vi "RT_Velocity mode_Oct 25.vi"() -> ()   [LabVIEW 2018]
uses:
  <vilib>/Platform/TimedLoop/XDataNode/XDataNode.xnode
  <vilib>/Platform/TimedLoop/XDataNode/nitl_modes.ctl
  <vilib>/Platform/TimedLoop/XDataNode/XDNodeRunTimeDep.lvlib
  <vilib>/Platform/TimedLoop/XDataNode/wakeup.ctl
  <vilib>/Platform/TimedLoop/XDataNode/timing_clust.ctl
  <vilib>/rvi/interface/nirviReadWriteControl/nirviReadWriteControl.xnode
  NiFpgaLv.dll
  <vilib>/Utility/error.llb/Error Cluster From Error Code.vi
  <vilib>/rvi/interface/Simulation/niFpgaSimulationCallBeginRW.vi
  <vilib>/rvi/errors/niLvFpgaAdjustHostInterfaceError.vi
  <vilib>/rvi/interface/nirviOpenFPGA/nirviOpenFPGA.xnode
  Type Defs/BL Measurement States.ctl
  <vilib>/rvi/interface/nirviCloseFPGA/nirviCloseFPGA.xnode
  <vilib>/FPGAPlugInAG/Dynamic/niLvFpga_Close_Dynamic.vi
  UNCC Watt balance Oct19/FPGA Bitfiles/UNCCWattbalanceO_FPGATarget_fpganestedFORW&R_sb-Oe1PDHtY.lvbitx
  FPGA files/fpga_nestedFOR_W&R_ADC_W_2DACs_Write_then_CLK.vi
  <vilib>/FPGAPlugInAG/myRIO-1900/niLvFpga_Open_myRIO-1900.vi
  <vilib>/rvi/interface/common/dynamic/niFpgaDynamicAddResources.vi
  <vilib>/addons/control/pid/NI_PID_pid.lvlib
  <vilib>/addons/control/pid/pid.llb/PID Lead-Lag (DBL).vi
panel:
  out "Velocity (m/s)":dbl=0.03333406380742028
  out "BL":dbl=14.310883864096947
  out "Cycles 2":dbl=2.5
  out "Time period 2":dbl=0.03704 format="%.4f"
  out "Amplitude (EMF)":dbl=0.47703991586638894 format="%.6f"
  out "Cycles":dbl=2.0
  out "Time period":dbl=0.037 format="%.4f"
  out "Amplitude (CP)":dbl=0.0001964918899367253 format="%.6f"
  in  "no. data points":u16=500
  in  "Measure":bool
  in  "Period (us)":i64=200
  in  "EMF Gain":dbl=1.0
  in  "offset (V)":dbl format="%#_13g"
  in  "frequency (Hz)":dbl=27.0 format="%#_13g"
  in  "amplitude (V)":dbl=0.4 format="%#_13g"
  out "Late? [i-1]":bool
  in  "Stop Button":bool
  out "?":cluster{dbl, dbl}(graph)={161.59573981109904, -162.80879503181404}
  out "sine fit debug":dbl[][](graph)=[[5.264201901216106e-07, 8.666859941712313e-06, 1.4091276683400212e-05, 2.2193570044402394e-05, 2.7587469673619477e-05, 3.5636358087797725e-05, 4.0946335657720054e-05, 4.886552634389733e-05, 5.410684041076032e-05, 6.187344553458349e-05, 6.953324076475882e-05, 7.45838228786792e-05, 8.20605154340296e-05, 8.694325342936049e-05, 9.181073286845596e-05, 9.892122007415655e-05, 0.00010359033828219172, 0.00011045668858812577, 0.00011494270412133601, 0.000121526771136915, 0.0001257915376047118, 0.0001320551749393472, 0.00013609869234173057, 0.00014198086577048074, 0.0001457726169949799, 0.00015131147290843336, 0.00015482857012069515, 0.00015994018645955715, 0.00016319788821581697, 0.00016785937714573442, 0.0001708500541678746, 0.00017506141568884748, 0.00017772403375192634, 0.00018147763858583694, 0.00018381982696797223, 0.0001871156751148206, 0.00018912980453789457, 0.000191906861772739, 0.0001936005615148694, 0.00019586645711582766, 0.0001978271815920777, 0.00019896394403161566, 0.00019994812090879955, 0.00020119169324198536, 0.00020184781116010795, 0.0002025573340250545, 0.00020285487587164497, 0.00020303797854646986, 0.00020299983215588135, 0.00020264125608434924, 0.000202259792178464, 0.00020139768375116338, 0.00020063475593939294, 0.00019926911515632384, 0.0001981857576636098, 0.00019629369669041909, 0.00019489753879487918, 0.00019249431618780224, 0.0001907395822207302, 0.00018787097364847332, 0.0001857958100004577, 0.00018243892762866772, 0.0001800433342997085, 0.00017622869524085627, 0.00017351267223095345, 0.00016924790576315664, 0.00016625722874101648, 0.0001615423348642751, 0.00015660619192212028, 0.00015315775821291784, 0.00014780200497428928, 0.00014409417580908492, 0.00014028716602835034, 0.00013441262187771787, 0.0001303614751972168, 0.0001241207256969345, 0.0001198407006729023, 0.00011328715076979413, 0.00010880113523658388, 0.00010191952637441442, 9.724277888826156e-05, 9.008651601385474e-05, 8.522666585287697e-05, 7.781863680058592e-05, 7.282145963348946e-05, 6.518455223766725e-05, 6.003478950821672e-05, 5.224529655004042e-05, 4.697346537070661e-05, 3.903901612829393e-05, 3.101301554846879e-05, 2.561148664113401e-05, 2.024047484627004e-05, 1.2100035094679337e-05, 6.6679890748737334e-06, -1.4800799548346732e-06, -6.919755252757983e-06, -1.5044936448113276e-05, -2.044646535544806e-05, -2.8472465935273197e-05, -3.377481422707782e-05, -4.166348780078428e-05, -4.685902619894104e-05, -5.456459709782259e-05, -5.962280848986067e-05, -6.71223888795642e-05, -7.20356439873659e-05, -7.928345819918517e-05, -8.404412774463277e-05, -9.10401757785678e-05, -9.56253719273082e-05, -0.00010233150739277047, -0.00010673360086668595, -0.00011311167737308692, -0.00011726963394723587, -0.00012332728077269324, -0.00012724872972519338, -0.00013294017120100092, -0.0001366327418099699, -0.0001419122022674214, -0.0001453148603079176, -0.00015019759830324852, -0.00015331797305338964, -0.00015774295436165825, -0.00016192379877016033, -0.00016455589972076836, -0.00016705067366525774, -0.00017056777087751953, -0.00017274974441918302, -0.000175770938553794, -0.0001776248531363962, -0.00018012725635900326, -0.00018163022414819104, -0.00018365198284938275, -0.0001848040038451561, -0.00018627645452187308, -0.00018710804583670288, -0.00018806170560141595, -0.0001885042037322428, -0.00018893144330683426, -0.00018904588247859982, -0.00018893144330683426, -0.0001886720478508323, -0.00018803881776706282, -0.00018742847551764645, -0.00018626882524375537, -0.0001853151654790423, -0.00018362146573691192, -0.00018232448845690216, -0.00018009673924653243, -0.00017846407372934368, -0.00017574805071944087, -0.0001737644384088377, -0.0001705525123212841, -0.00016824847032973733, -0.00016455589972076836, -0.00016193905732639571, -0.00015778110075224678, -0.00015485145795504824, -0.00015026626180630786, -0.00014706196499687194, -0.00014201901216106928, -0.00013854769061751374, -0.00013313090315394355, -0.00012940018615438602, -0.0001235866762286952, -0.00011962708088560657, -0.00011345499488838362, -0.00010925126264552846, -0.00010278926407983273, -9.835665349344641e-05, -9.158948380304253e-05, -8.698139981994901e-05, -7.992431756107234e-05, -7.513313090315393e-05, -6.7824282466393e-05, -6.287288096800279e-05, -5.5342783465828454e-05, -4.768298823565312e-05, -4.2525596228084886e-05, -3.467506904496696e-05, -2.941086714375085e-05, -2.1438271510749647e-05, -1.6067259715885676e-05, -1.06809893647863e-05, -2.5786960037841213e-06, 2.8304621816683697e-06, 1.0963272655141367e-05, 1.639531867494697e-05, 2.4482353479713745e-05, 3.253887117200969e-05, 3.789462441063825e-05, 4.319697270244288e-05, 5.110090483238475e-05, 5.631933106489462e-05, 6.404016052001157e-05, 6.916703541510901e-05, 7.672765002975416e-05, 8.167905152814438e-05, 8.903367563361153e-05, 9.385537940400076e-05, 0.00010094297877534824, 0.00010558920914903028, 0.00011242504234249352, 0.00011686528220699753, 0.00012338831499763487, 0.00012972061583532962, 0.00013380990890641924, 0.0001378229091963318, 0.00014365167767825806, 0.00014741291179028634, 0.00015286784564444507, 0.00015636205502235373, 0.000161389749301921, 0.0001646016753894746, 0.0001691792422600973, 0.00017210888505729584, 0.00017625921235332707, 0.00017885316691334662, 0.00018253047896608018, 0.00018483452095762693, 0.00018800067137647431, 0.00018997665440895979, 0.00019266216030639174, 0.0001942795672673451, 0.00019646917008712627, 0.00019774325953278294, 0.00019941407144056023, 0.00020036010192715559, 0.00020151975220104667, 0.0002020995773379922, 0.00020272517814364397, 0.00020296168576529282, 0.00020305323710270528, 0.00020280910020293872, 0.0002017410012664601, 0.0002010848833483375, 0.00020026855058974312, 0.00019879609991302617, 0.00019765170819537048, 0.0001956528373285319, 0.00019416512809557955, 0.00019168561270732555, 0.00018987747379342962, 0.00018687916749317174, 0.0001847658574545676, 0.00018130979446724746, 0.0001788455376352289, 0.00017493934723896419, 0.00017220043639470828, 0.0001678288600332636, 0.00016480003662053491, 0.00015999359140638107, 0.00015666722614706192, 0.00015147931702702284, 0.00014787829775546633, 0.00014231655400765976, 0.0001384713978363367, 0.00013252056090452718, 0.00012845415566779066, 0.00012212185483009594, 0.0001178189419717106, 0.00011120435784366079, 0.00010668019591986203, 9.976044066710405e-05, 9.504554679036267e-05, 8.784350824724962e-05, 8.294551169568333e-05, 7.551459480903914e-05, 7.047927125135417e-05, 6.282710529929656e-05, 5.7646825457375206e-05, 4.9834444664845795e-05, 4.455498420739428e-05, 3.6597647130628485e-05, 3.1219006057646816e-05, 2.3147229809115453e-05, 1.7753330179898374e-05, 9.605261150189966e-06, 4.196102964737475e-06, -3.944336786853227e-06, -9.361124250423422e-06, -1.7486305445778715e-05, -2.2842058684407274e-05, -3.08604299861147e-05, -3.8764362116056565e-05, -4.397515907044874e-05, -4.915543891237009e-05, -5.680760486442771e-05, -6.435296092283746e-05, -7.659795230175319e-05, -8.13967682377893e-05, -8.844622121854828e-05, -9.304667592352409e-05, -9.759372568167598e-05, -0.00010425408547843201, -0.00010858751544928816, -0.0001149350748432183, -0.00011905488502677873, -0.00012505149762729448, -0.00012893480018920606, -0.00013454994888383655, -0.0001381585974335108, -0.0001434151700566092, -0.00014674153531592837, -0.00015154798053008218, -0.0001546225796115171, -0.0001590017852510795, -0.00016175595465157082, -0.0001656545157697178, -0.00016811877260173636, -0.0001715443184765857, -0.00017366525779330755, -0.00017661015914674147, -0.00017842592733875517, -0.00018084440850206748, -0.00018298060637502475, -0.0001842546958206814, -0.00018535331186963084, -0.00018678761615575928, -0.00018753528541129433, -0.00018841265239483035, -0.0001888398919694218, -0.0001891908387628362, -0.00018924424370966015, -0.00018908402886918835, -0.00018877885774448017, -0.00018806933487953365, -0.00018743610479576416, -0.00018622304957504915, -0.00018520835558539446, -0.00018346888017455783, -0.00018213375650395953, -0.00017985260234676587, -0.00017819704899522403, -0.00017541236248226188, -0.000173421120893541, -0.00017015578985916347, -0.00016781360147702818, -0.000164075255199353, -0.00016142026641439183, -0.00015723179272777204, -0.00015429452065245582, -0.0001496559195568915, -0.00014642873491310248, -0.0001413781527991821, -0.00013609106306361287, -0.00013242138028899701, -0.00012675282664754257, -0.00012286952408563096, -0.00011886415307383611, -0.00011268443779849546, -0.00010847307627752259, -0.00010201107771182688, -9.757083784732285e-05, -9.078078032256585e-05, -8.617269633947233e-05, -7.910798480247797e-05, -7.433205670079494e-05, -6.701557898591633e-05, -6.208706532187922e-05, -5.4526450707234066e-05, -4.946061003707828e-05, -4.172452202572591e-05, -3.649846651509833e-05, -2.8617422219509583e-05, -2.3322703205822658e-05, -1.5296702625997522e-05, -9.93332010925126e-06, -1.8386560263667845e-06, 0.0, 0.0, 0.0, 0.0, 0.0, 0.0, 0.0, 0.0, 0.0, 0.0, 0.0, 0.0, 0.0, 0.0, 0.0, 0.0, 0.0, 0.0, 0.0, 0.0, 0.0, 0.0, 0.0, 0.0, 0.0, 0.0, 0.0, 0.0, 0.0, 0.0, 0.0, 0.0, 0.0, 0.0, 0.0, 0.0, 0.0, 0.0, 0.0, 0.0, 0.0, 0.0, 0.0, 0.0, 0.0, 0.0, 0.0, 0.0, 0.0, 0.0, 0.0, 0.0, 0.0, 0.0, 0.0, 0.0, 0.0, 0.0, 0.0, 0.0, 0.0, 0.0, 0.0, 0.0, 0.0, 0.0, 0.0, 0.0, 0.0, 0.0, 0.0, 0.0, 0.0, 0.0, 0.0, 0.0, 0.0, 0.0, 0.0, 0.0, 0.0, 0.0, 0.0, 0.0, 0.0, 0.0, 0.0, 0.0, 0.0, 0.0, 0.0, 0.0, 0.0], [-0.00167844118589499, -0.01953095198132352, -0.03860414727558477, -0.050505821139203794, -0.05508338800982649, -0.07491951111585819, -0.09704441765720125, -0.10787799258434164, -0.12389947663152108, -0.14236232967636597, -0.15502693135175544, -0.16357172284358448, -0.181424233639013, -0.19485176312617294, -0.21239910279689328, -0.22628438897111547, -0.24062743183239993, -0.24962998001129125, -0.26626180630788704, -0.2789264079832765, -0.2900651540351251, -0.30028838671284913, -0.31661504188473677, -0.3251598333765658, -0.3388925339884339, -0.34774249660497114, -0.35994934159329833, -0.3694096464592519, -0.3796328791369759, -0.38894059844057544, -0.40084227230419445, -0.40648793811129574, -0.415337900727833, -0.4211361520972884, -0.4286128446526388, -0.44005676182919556, -0.4457024276362969, -0.4495170666951491, -0.4592825426858109, -0.45867220043639456, -0.4672169919282236, -0.4688954331141186, -0.47225231548590857, -0.474693684483574, -0.47972900804125895, -0.4774402246059476, -0.4856798449730685, -0.48323847597540304, -0.4791186657918426, -0.4841539893495276, -0.4803393502906753, -0.4772876390435935, -0.474693684483574, -0.4734729999847413, -0.4681325053023481, -0.4600454704975814, -0.4595877138105191, -0.4545523902528341, -0.4481437966339623, -0.44036193295390375, -0.4333429970856156, -0.42342493553259974, -0.41472755847841664, -0.4106077482948562, -0.39748538993240445, -0.39092421075117856, -0.3779544379510809, -0.3625432961533178, -0.3523200634755938, -0.3416390741108075, -0.32729603124952306, -0.32393914887773306, -0.3082228359552618, -0.2938797930939773, -0.2766376245479652, -0.26290492393609705, -0.2503929078230617, -0.23910157620885902, -0.22231716434990914, -0.21011031936158192, -0.19134229519202886, -0.18249233257549163, -0.16540274959183357, -0.1512122922929032, -0.13015548468803878, -0.11825381082441976, -0.10452111021255166, -0.08514274379358222, -0.06561179181225871, -0.05721958588278375, -0.03753604833910614, -0.02212490654134305, -0.00946030486595358, 0.0076292781177045, 0.02990677022140164, 0.03997741733677158, 0.0564566580710133, 0.0701893586828814, 0.08300654592062497, 0.09872285884309623, 0.11184521720554798, 0.12771411569037333, 0.1388528617422219, 0.15929932709766997, 0.1815768192013671, 0.18981643956848795, 0.20721119367685423, 0.21865511085341097, 0.22811541571936456, 0.24383172864183583, 0.25405496131955985, 0.27083937317850976, 0.28609792941391876, 0.2941849642186855, 0.3076124937058454, 0.3199719242565267, 0.33065291362131305, 0.3434701008590566, 0.3539985046614888, 0.36376398065215054, 0.3761234112028319, 0.3861940583182018, 0.39626470543357173, 0.40786120817248256, 0.41793185528785254, 0.4189999542243312, 0.42784991684086837, 0.435784366083281, 0.44341364420098556, 0.4498222378198573, 0.45577307475166684, 0.46599630742939085, 0.46904801867647267, 0.46935318980118085, 0.47393075667180357, 0.4771350534812394, 0.48171262035186213, 0.48629018722248485, 0.4855272594107144, 0.4858324305354226, 0.4872057005966094, 0.4833910615377571, 0.4826281337259867, 0.4821703770389244, 0.4804919358530294, 0.47652471123182305, 0.4731678288600331, 0.47118421654942994, 0.46630147855409904, 0.45867220043639456, 0.4519584356928146, 0.44539725651158873, 0.440819689640966, 0.43166455589972064, 0.42357752109495383, 0.41442238735370845, 0.40496208248775484, 0.39779056105711263, 0.3893983551276377, 0.3767337534522482, 0.36544242183804554, 0.3541510902238429, 0.34270717304728615, 0.32866930131070987, 0.31890382532004813, 0.3039504402093473, 0.29525306315516414, 0.27953675023269287, 0.2670247341196575, 0.24993515113599943, 0.23223522590292497, 0.2229275065993255, 0.2061430947403756, 0.19515693425088113, 0.18081389138959666, 0.16463982178006312, 0.1449562842363855, 0.13320719593512056, 0.11047194714436116, 0.10284266902665666, 0.08743152722889357, 0.07385141217937956, 0.05630407250865921, 0.03692570608968978, 0.03021194134610982, 0.00839220592947495, -0.00976547599066176, -0.01998870866838579, -0.03570502159085706, -0.05599890138395103, -0.06439110731342598, -0.08697377054183131, -0.09521339090895216, -0.11077711826906934, -0.13229168256099602, -0.14159940186459552, -0.1574683003494209, -0.17669408120603622, -0.1889009261943634, -0.19805605993560882, -0.2091948059874574, -0.2239956055358041, -0.24139035964417038, -0.2564963303172253, -0.26900834643026067, -0.27984192135740105, -0.2928116941574987, -0.30562888139524225, -0.3181408975082777, -0.32744861681187715, -0.3422494163602239, -0.3495735233532202, -0.3642217373392128, -0.37337687108045825, -0.37902253688755955, -0.3906190396264704, -0.40053710117948627, -0.4104551627325021, -0.4167111707890198, -0.42525596228084883, -0.43013870027617973, -0.4379205639562383, -0.44753345438454595, -0.4511955078810441, -0.45714634481285366, -0.46050322718464365, -0.46035064162228956, -0.4702687031753054, -0.4719471443612004, -0.47560919785769856, -0.47652471123182305, -0.47576178342005265, -0.48171262035186213, -0.4771350534812394, -0.47805056685536396, -0.47652471123182305, -0.4748462700459281, -0.47454109892121993, -0.47072645986236766, -0.46736957749057767, -0.4650807940552663, -0.4623342539328927, -0.45562048918931275, -0.4487541388833787, -0.43700505058211375, -0.43669987945740557, -0.4309016280879502, -0.4228145932831834, -0.4133542884172298, -0.3968750476829881, -0.39412850756061446, -0.38192166257228727, -0.37352945664281234, -0.3619329539039015, -0.34804766772967927, -0.33614599386606026, -0.32088743763065125, -0.3066969803317209, -0.30517112470818003, -0.2883867128492301, -0.2682454186184902, -0.25741184369134984, -0.24078001739475402, -0.22719990234524, -0.22048613760166005, -0.20110777118269063, -0.19164746631673704, -0.1708958298365808, -0.1541114179776309, -0.13656407830691056, -0.12252620657033426, -0.10665730808550891, -0.09750217434426352, -0.07385141217937956, -0.06271266612753099, -0.04318171414620747, -0.02609213116254939, -0.01159650273891084, 0.00656117918122587, 0.02090422204251033, 0.03265331034377526, 0.0518790912003906, 0.06347559393930144, 0.0825487892335627, 0.09490821978424398, 0.11230297389261024, 0.1266460167538947, 0.1420571585516578, 0.1599096693470863, 0.18722248500846844, 0.20095518562033654, 0.21682408410516188, 0.22796283015701047, 0.24322138639241947, 0.25390237575720576, 0.2673299052443657, 0.28014709248210923, 0.29098066740924966, 0.3083754215176159, 0.31692021300944495, 0.3298899858095426, 0.33782443505195525, 0.3527778201626561, 0.35949158490623606, 0.37505531226635325, 0.3826845903840577, 0.396722462120634, 0.4031310557395058, 0.4121336039183971, 0.4167111707890198, 0.43120679921265836, 0.43547919495857285, 0.4457024276362969, 0.44936448113279504, 0.45531531806460457, 0.4620290828081845, 0.4669118208035154, 0.4731678288600331, 0.48156003478950804, 0.48171262035186213, 0.4870531150342553, 0.4840014037871735, 0.4836962326624653, 0.4858324305354226, 0.48766345728367166, 0.49315653752841887, 0.49178326746723205, 0.48476433159894394, 0.4836962326624653, 0.47972900804125895, 0.4760669545447608, 0.47682988235653123, 0.4714893876741381, 0.4698109464882431, 0.4609609838717059, 0.4533317057540014, 0.4440239864504019, 0.44158261745273647, 0.4275447457161602, 0.4208309809725802, 0.41274394616781346, 0.39931641668065354, 0.39397592199826037, 0.38253200482170363, 0.3623907105909637, 0.35140455010146926, 0.3370615072401848, 0.32897447243541805, 0.30517112470818003, 0.3004409722752032, 0.2868608572256892, 0.2734333277385293, 0.26427819399728386, 0.24749378213833398, 0.2365076216488395, 0.22201199322520096, 0.2076689503639165, 0.18981643956848795, 0.1768466667683903, 0.16052001159650267, 0.14693989654698866, 0.1300028991256847, 0.11642278407617067, 0.10040130002899122, 0.08697377054183131, 0.06851091749698641, 0.05721958588278375, 0.03829897615087659, 0.02471886110136258, 0.0045775668706227, -0.01480079954834673, -0.02670247341196575, -0.04211361520972884, -0.05569373025924285, -0.06652730518638324, -0.0884996261653722, -0.09780734546897168, -0.12237362100798019, -0.12588308894212424, -0.14739765323405093, -0.15624761585058816, -0.17165875764835126, -0.1879854128202389, -0.2046172391168347, -0.21484047179455873, -0.2316248836535086, -0.23559210827471497, -0.2529868623830812, -0.26794024749378204, -0.28152036254329604, -0.2955582342798723, -0.3066969803317209, -0.32088743763065125, -0.3315684269954376, -0.34301234417199433, -0.35445626134855107, -0.364526908463921, -0.3724613577063337, -0.3883302561911591, -0.3935181653111981, -0.4035888124265681, -0.4118284327936889, -0.4208309809725802, -0.4258663045302652, -0.43288524039855336, -0.44341364420098556, -0.44905931000808685, -0.4515006790057523, -0.45729893037520775, -0.4632497673070172, -0.46752216305293176, -0.4699635320505972, -0.4731678288600331, -0.4753040267329904, -0.47942383691655077, -0.47988159360361304, -0.48110227810244577, -0.4838488182248194, -0.48171262035186213, -0.4821703770389244, -0.4792712513541967, -0.4748462700459281, -0.47454109892121993, -0.4685902619894104, -0.4634023528693713, -0.4620290828081845, -0.45729893037520775, -0.45241619237987685, -0.4460075987610051, -0.43410592489738603, -0.42983352915147155, -0.42006805316080975, -0.411981018356043, -0.4032836413018599, -0.39458626424767673, -0.3843630315699527, -0.37520789782870734, -0.3587286570944656, -0.3539985046614888, -0.34255458748493206, -0.3295848146848344, -0.3176831408212154, -0.3004409722752032, -0.2851824160397942, -0.27617986786090293, -0.259395456001953, -0.2429162152677113, -0.23757572058531815, -0.22094389428872233, -0.20385431130506423, -0.18508628713551117, -0.16998031646245626, -0.1618932816576895, -0.1437355997375528, -0.13534339380807783, -0.10955643377023662, -0.09338236416070309, -0.08010742023589724, -0.05996612600515737, -0.04775928101683017, -0.0396722462120634, -0.015258556235409, -0.0030517112470818]]
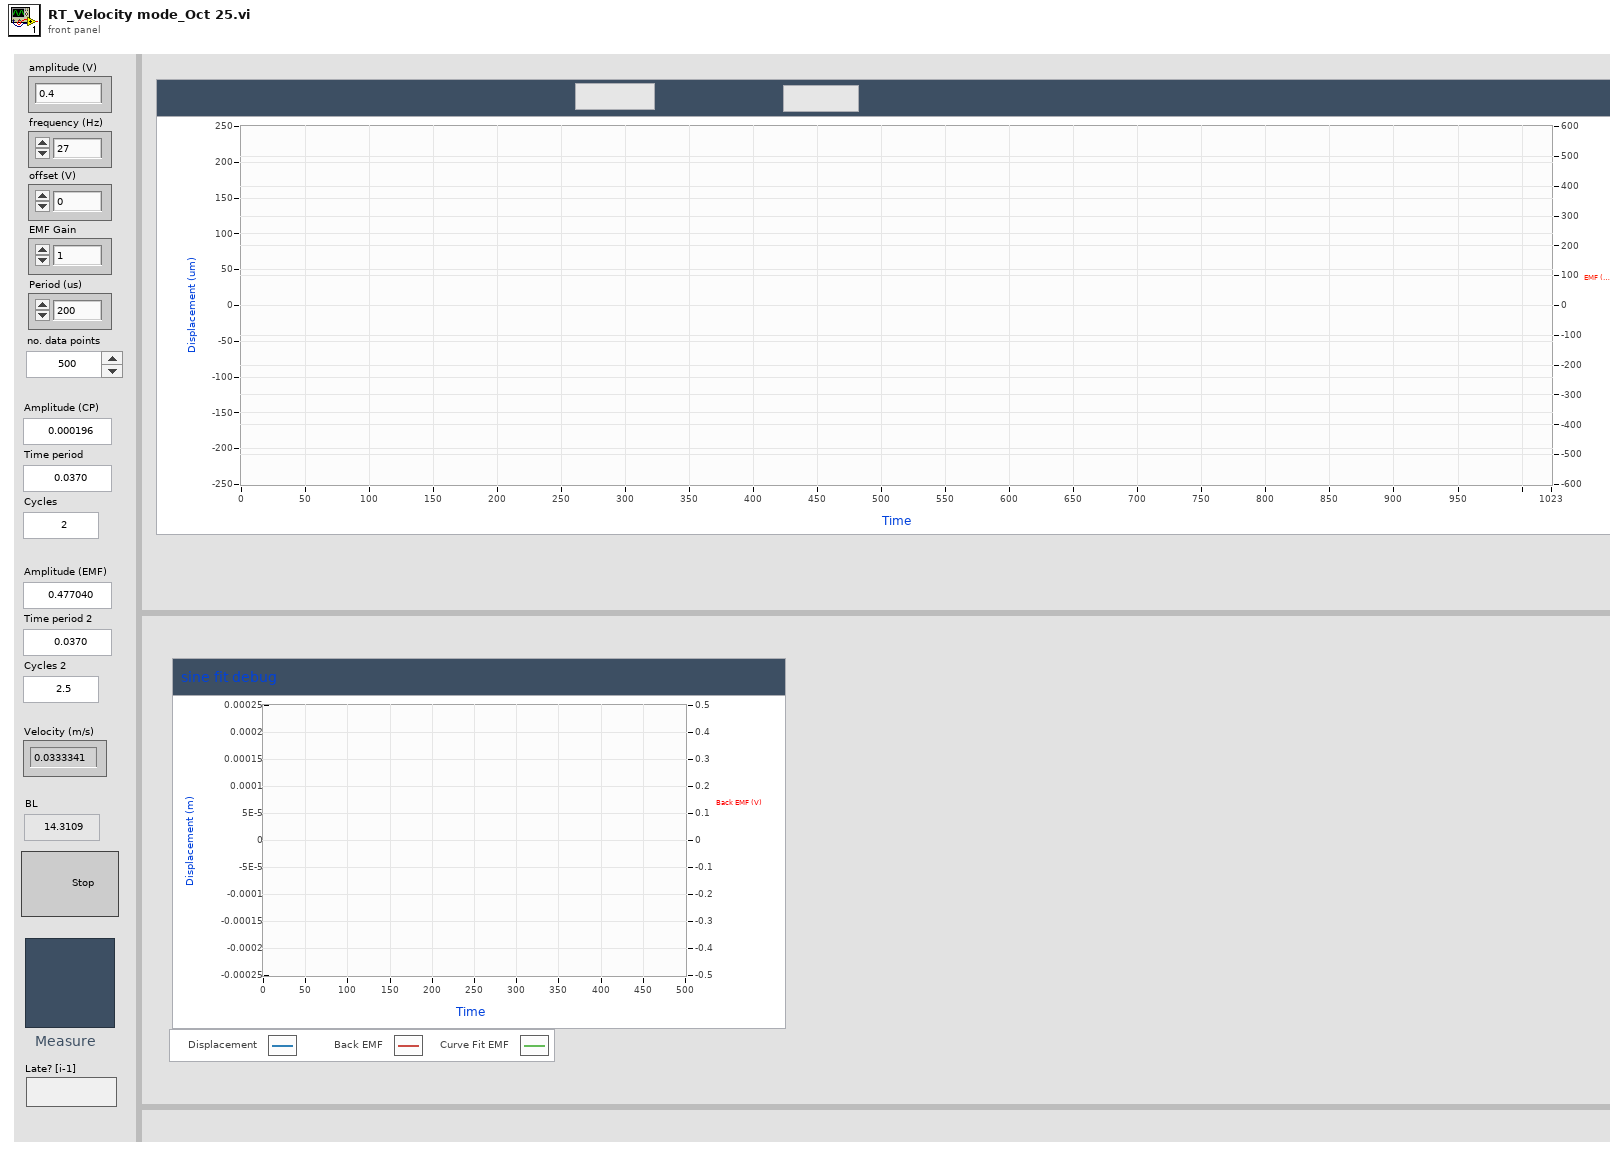
[diagram p1: front panel]
types:
  T1 = typedef "BL Measurement States.ctl" = enum16{"reset BL avg", "idle", "initialize", "collect data", "prepare data", "fit sine", "calculate BL", "exit meas"}
  T2 = typedef "XDNodeRunTimeDep.lvlib/timing_clust.ctl" = cluster{"Expected End [f-1]":u64, "Actual End [f-1]":u64, "Finished Late? [f-1]":bool, "Expected End [i-1]":u64, "Actual End [i-1]":u64, "Finished Late? [i-1]":bool, "Expected Start [i]":u64, "Actual Start [i]":u64, "Expected Start [f]":u64, "Actual Start [f]":u64, "Source Name":string, "Structure Name":string, "Period":i64, "Deadline":i64, "Offset":i64, "Start":i64, "Priority":i32, "Timeout":i32, "Mode":T3, "Wakeup Reason":T4, "Error":errorcluster, "Source Type":string, "Secondary Source Type":string, "Global End Time":u64, "Global Start Time":u64, "Frame Duration":u64, "Iteration Duration":u64, "Assigned CPU":i32, "I/O Scan Engine Mode":u32}
  T3 = typedef "XDNodeRunTimeDep.lvlib/nitl_modes.ctl" = enum32{"No Change", "Process missed periods, maintain original phase", "Discard missed periods, maintain original phase", "Process missed periods, ignore original phase", "Discard missed periods, ignore original phase"}
  T4 = typedef "XDNodeRunTimeDep.lvlib/wakeup.ctl" = enum32{"Normal", "Aborted", "Asynchronous wakeup", "Timing source error", "Timed loop error", "Timeout"}
  T5 = typedef "Fourier Outputs.ctl" = cluster{"Time period":dbl, "computed \namplitude":dbl, "number of cycles":dbl}
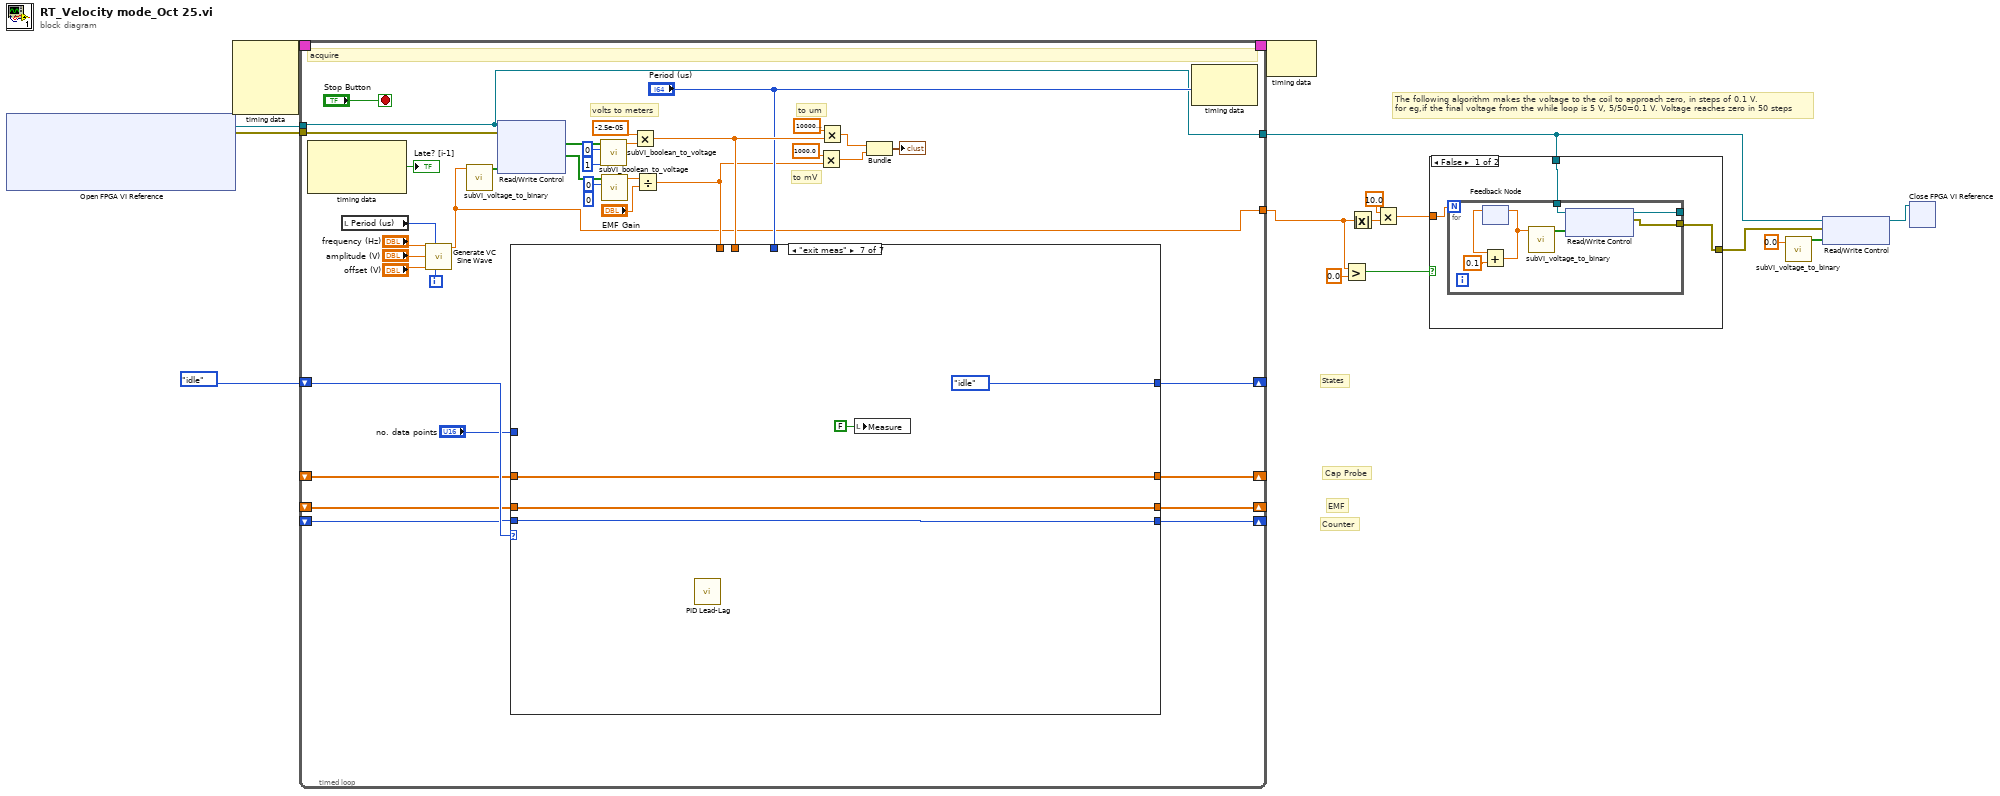
[diagram p0: block diagram]
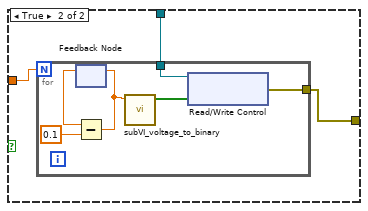
[diagram p2: hidden frame]
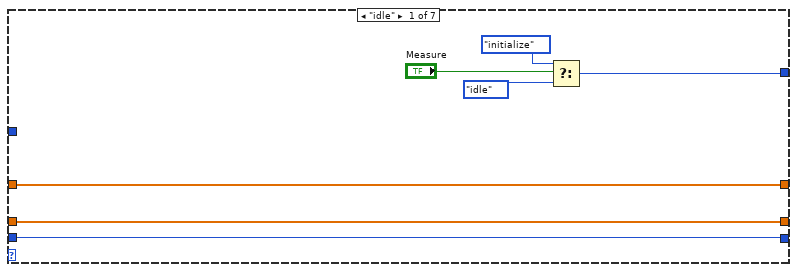
[diagram p3: hidden frame]
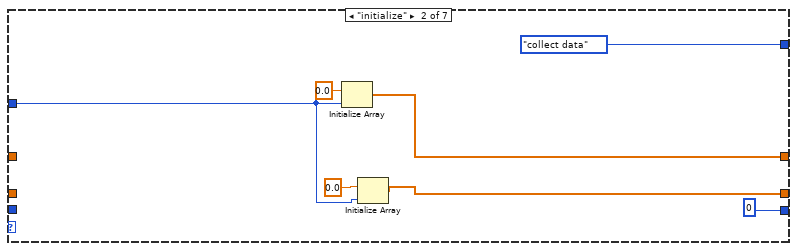
[diagram p4: hidden frame]
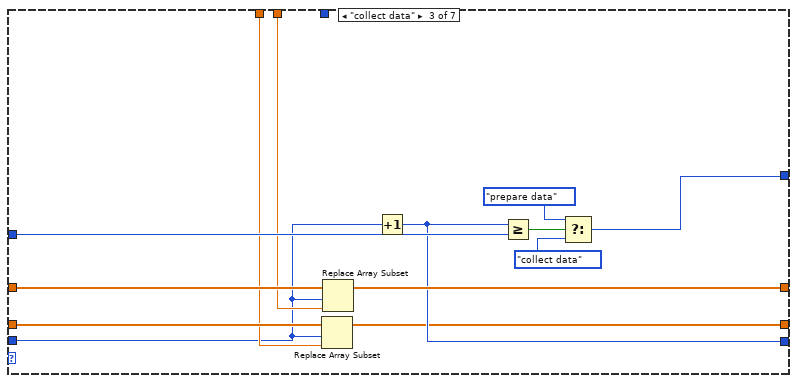
[diagram p5: hidden frame]
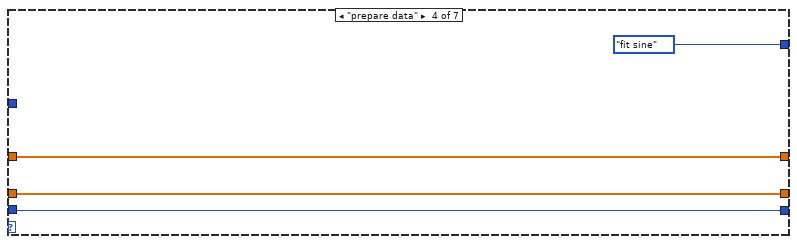
[diagram p6: hidden frame]
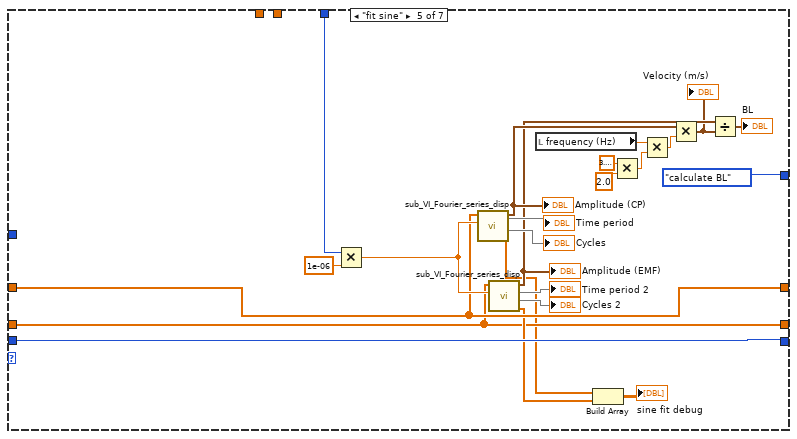
[diagram p7: hidden frame]
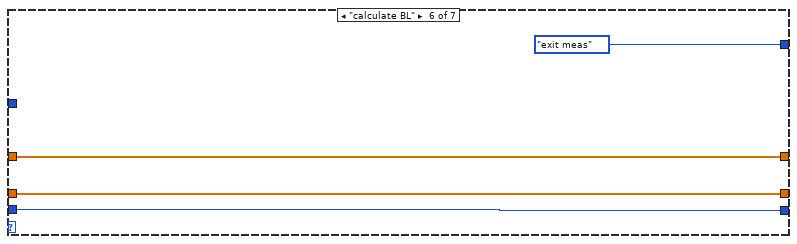
[diagram p8: hidden frame]
diagram:
  # "The following algorithm makes the voltage to the coil to approach zero, in steps of 0.1 V.\nfor eg,if the final voltage from the while loop is 5 V, 5/50=0.1 V. Voltage reaches zero in 50 steps"
  # "States"
  # "Counter"
  # "EMF"
  # "Cap Probe"
  n1 = xnode "Open FPGA VI Reference"() -> ("FPGA VI Reference Out"=w14:refnum<k20>, "error out"=w13:errorcluster)  [unwired: 2 in]
  n2 = node-c288() -> (w16:T2)  [unwired: 4 in]
  n3 = timed-loop {
    timing: w16 -> [_]
    timing-out: [_] -> w15
    tunnel: w14 -> [w17]
    tunnel: w13 -> [w44]
    shift-right: [w37] -> _
    shift-left: BL_Measurement_States."idle" ("BL meas states") -> [w38]
    shift-right: [w36] -> _
    shift-left: _ -> [w35]
    shift-right: [w33] -> _
    shift-left: _ -> [w34]
    shift-right: [w25] -> _
    shift-left: _ -> [w26]
    tunnel: [w18] -> w2
    tunnel: [w17] -> w1
    i -> [w53]
    stop <- "Stop Button" stop-if-true
    (unwired) i16 0 ("Gain")
    # "to mV"
    # "to um"
    # "volts to meters"
    # "acquire"
    n4 = node-c288() -> (→"Late? [i-1]":bool)  [unwired: 1 in, 2 out]
    n5 = local read "Period (us)"() -> (w48:i64)
    n6 = call "Generate VC Sine Wave.vi"("Counter"=w53, "Period (us)"=w48, "offset (V)"="offset (V)", "amplitude (V)"="amplitude (V)", "frequency (kHz)"="frequency (Hz)") -> ("V"=w18:dbl)  [unwired: 6 in]
    n7 = call "subVI_voltage_to_binary.vi"("voltage"=w18) -> ("binary"=w45:bool[])  [unwired: 10 in]
    n8 = xnode "Read/Write Control"("FPGA VI Reference In"=w17, "error in"=w44, "DAC 1 write"=w45) -> ("ADC  1 R"=w40:bool[], "ADC 2 R"=w39:bool[])  [unwired: 2 out]
    n9 = call "subVI_boolean_to_voltage.vi"("Gain"=i16 1, "UNI"=i16 0, "ADC read"=w40) -> ("V"=w32:dbl)  [unwired: 8 in]
    n10 = call "subVI_boolean_to_voltage.vi"("UNI"=i16 0, "ADC read"=w39) -> ("V"=w31:dbl)  [unwired: 9 in]
    n11 = Multiply(x=-2.5e-05, y=w32) -> (x*y=w30:dbl)
    n12 = Divide(x=w31, y="EMF Gain") -> (x/y=w27:dbl)
    n13 = case shown="\"exit meas\"" w38 {
      tunnel: [w58 BL_Measurement_States."collect data" ("BL meas states") w74 BL_Measurement_States."fit sine" ("BL meas states") BL_Measurement_States."calculate BL" ("BL meas states") BL_Measurement_States."exit meas" ("BL meas states") BL_Measurement_States."idle" ("BL meas states")] -> w37
      tunnel: [w55 w63 w75 w82 w90 w110 w115] -> w36
      tunnel: [w54 w62 w70 w81 w87 w108 w112] -> w25
      tunnel: w35 -> [w55 _ w77 w82 w90 w110 w115]
      tunnel: w34 -> [w56 _ w68 w84 w107 w109 w114]
      tunnel: [w56 0 w72 w84 w107 w109 w114] -> w33
      tunnel: "no. data points" -> [_ w61 w76 _ _ _ _]
      tunnel: w30 -> [_ _ w73 _ _ _ _]
      tunnel: "Period (us)" -> [_ _ _ _ w104 _ _]
      tunnel: w27 -> [_ _ w69 _ _ _ _]
      tunnel: w26 -> [w54 _ w71 w81 w87 w108 w112]
      frame "idle" {
        n14 = Select(t=BL_Measurement_States."initialize" ("BL meas states"), s="Measure", f=BL_Measurement_States."idle" ("BL meas states 2")) -> (s? t:f=w58:T1)
      }
      frame "initialize" {
        n15 = Initialize Array(0.0 ("element"), w61) -> (w63:dbl[])
        n16 = Initialize Array(0.0 ("element"), w61) -> (w62:dbl[])
      }
      frame "collect data" {
        n17 = Replace Array Subset(array=w71, new element=w69, index=w68) -> (w70:dbl[])
        n18 = Replace Array Subset(array=w77, new element=w73, index=w68) -> (w75:dbl[])
        n19 = Increment(x=w68) -> (x+1=w72:i32)
        n20 = Greater Or Equal?(x=w72, y=w76) -> (x >= y?=w78:bool)
        n21 = Select(t=BL_Measurement_States."prepare data" ("BL meas states"), s=w78, f=BL_Measurement_States."collect data" ("BL meas states 2")) -> (s? t:f=w74:T1)
      }
      frame "prepare data" {
      }
      frame "fit sine" {
        n22 = Multiply(x=w104, y=1e-06) -> (x*y=w92:dbl)
        n23 = call "sub_VI_Fourier_series_disp.vi"("del t"=w92, "x,i"=w90) -> ("clipped array"=w85:dbl[], 1:→"Cycles", 2:→"Time period", "outputs"=w99:T5)  [unwired: 6 in]
        "Amplitude (CP)" <- w99
        n24 = call "sub_VI_Fourier_series_disp.vi"("del t"=w92, "x,i"=w87) -> ("clipped array"=w88:dbl[], 1:→"Cycles 2", 2:→"Time period 2", "outputs"=w91:T5)  [unwired: 6 in]
        "Amplitude (EMF)" <- w91
        n25 = local read "frequency (Hz)"() -> (w93:dbl)
        n26 = Build Array(w85, w88) -> (→"sine fit debug":dbl[][])
        n27 = Multiply(x=3.141592653589793, y=2.0) -> (x*y=w97:dbl)
        n28 = Multiply(x=w93, y=w97) -> (x*y=w94:dbl)
        n29 = Multiply(x=w99, y=w94) -> (x*y=w86:T5)
        "Velocity (m/s)" <- w86
        n30 = Divide(x=w91, y=w86) -> (x/y=→"BL":T5)
      }
      frame "calculate BL" {
      }
      frame "exit meas" {
        n31 = call-poly <vilib>:"PID Lead-Lag.vi"() -> ()  [unwired: 8 in, 2 out]
        n32 = local write "Measure"(FALSE) -> ()
      }
    }
    n33 = Multiply(x=1000.0, y=w27) -> (x*y=w21:dbl)
    n34 = Multiply(x=1000000.0, y=w30) -> (x*y=w19:dbl)
    n35 = Bundle(w19, w21) -> (→"?":cluster{dbl, dbl})  [unwired: 1 in]
    n36 = node-c288("Period (us)") -> ()  [unwired: 1 in, 1 out]
  }
  n37 = node-c288(w15) -> ()  [unwired: 1 out]
  n38 = Greater?(x=w2, y=0.0) -> (0:w11:bool)
  n39 = Absolute Value(x=w2) -> (abs(x)=w7:dbl)
  n40 = Multiply(x=10.0, y=w7) -> (x*y=w10:dbl)
  n41 = case shown="False" w11 {
    tunnel: w10 -> [w124 w134]
    tunnel: w1 -> [w123 w133]
    tunnel: [w122 w132] -> w3
    frame False {
      n42 = for {
        N: w124 -> [_]
        tunnel: [w130] -> _
        tunnel: [w126] -> w122
        tunnel: w123 -> [w125]
        n43 = feedback #1() -> (w128:dbl)  [unwired: 1 in]
        n44 = Add(x=w128, y=0.1) -> (x+y=w127:dbl)
        n45 = feedback-in #1(w127) -> ()
        n46 = call "subVI_voltage_to_binary.vi"("voltage"=w127) -> ("binary"=w131:bool[])  [unwired: 10 in]
        n47 = xnode "Read/Write Control"("FPGA VI Reference In"=w125, "DAC 1 write"=w131) -> ("FPGA VI Reference Out"=w130:refnum<k20>, "error out"=w126:errorcluster)  [unwired: 1 in]
      }
    }
    frame True {
      n48 = for {
        N: w134 -> [_]
        tunnel: [w136] -> w132
        tunnel: w133 -> [w135]
        n49 = feedback #2() -> (w139:dbl)  [unwired: 1 in]
        n50 = Subtract(x=w139, y=0.1) -> (x-y=w137:dbl)
        n51 = feedback-in #2(w137) -> ()
        n52 = call "subVI_voltage_to_binary.vi"("voltage"=w137) -> ("binary"=w140:bool[])  [unwired: 10 in]
        n53 = xnode "Read/Write Control"("FPGA VI Reference In"=w135, "DAC 2 write"=w140) -> ("error out"=w136:errorcluster)  [unwired: 1 in, 1 out]
      }
    }
  }
  n54 = call "subVI_voltage_to_binary.vi"("voltage"=0.0) -> ("binary"=w5:bool[])  [unwired: 10 in]
  n55 = xnode "Read/Write Control"("FPGA VI Reference In"=w1, "error in"=w3, "DAC 1 write"=w5) -> ("FPGA VI Reference Out"=w6:refnum<k20>)  [unwired: 1 out]
  n56 = xnode "Close FPGA VI Reference"("FPGA VI Reference In"=w6) -> ()  [unwired: 1 in, 1 out]
